vi "Resize_RetainData_Greyscale.vi"(8 "error in (no error)":errorcluster, 9 "OpenCV Interpolation Flag":T1, 10 "New Image Size":T2, 11 "Greyscale Image":refnum<data-value>) -> (0 "error out":errorcluster, 3 "Greyscale Image (duplicate)":refnum<data-value>)   [LabVIEW 2020, in "g_ar_toolkit.lvlib"]
uses:
  g_ar_toolkit.lvlib
  Image Size Cluster.ctl
  OpenCV Interpolation Enum.ctl
  <vilib>/Utility/error.llb/Error Cluster From Error Code.vi
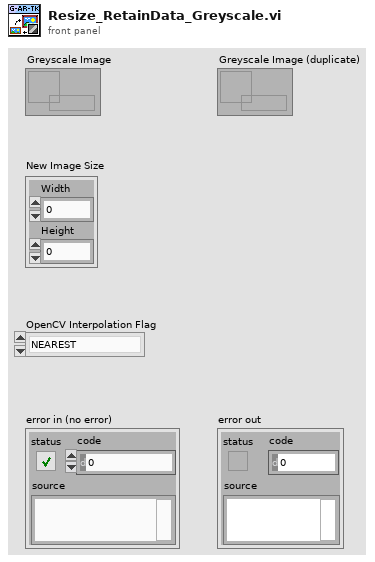
[diagram p1: front panel]
types:
  T1 = typedef "g_ar_toolkit.lvlib/OpenCV Interpolation Enum.ctl" = enum16{"NEAREST", "LINEAR", "CUBIC", "AREA", "LANCZOS", "LINEAR_EXACT", "NEAREST_EXACT", "MAX"}
  T2 = typedef "g_ar_toolkit.lvlib/Image Size Cluster.ctl" = cluster{"Width":u16, "Height":u16}
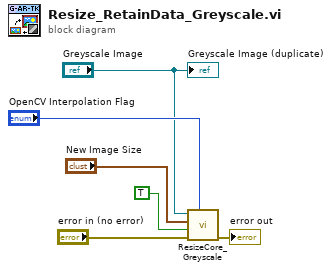
[diagram p0: block diagram]
diagram:
  n1 = call "ResizeCore_Greyscale.vi"("OpenCV Interpolation Flag"="OpenCV Interpolation Flag", "error in (no error)"="error in (no error)", "Retain Data?"=TRUE, "ImageSize"="New Image Size", "Greyscale Image"="Greyscale Image") -> ("error out"=→"error out":errorcluster)  [unwired: 6 in]
  "Greyscale Image (duplicate)" <- "Greyscale Image"
